vi "Read Glimpse simple.vi"() -> ()   [LabVIEW 2014]
uses:
  4.Other/header ctl/Header file data.ctl
  4.Other/header ctl/Offset table.ctl
  4.Other/header ctl/Offset.ctl
  4.Other/header ctl/file number.ctl
panel:
  out "Header file data":T1 {"Pixel depth" items=["8 bits", "16 bits", "Float", "Complex", "RGB", "HSL"]; "time of 1st frame, \nsec since 1/1/04" format="%.2f"}
  out "size(s)":i32
  out "TTB Array (ms)":u32[](array[numeric])
  out "Array":u32[](array[numeric])
  in  "Data Folder":path
  out "Image":T5(plugin-control)
  out "Width":i32=1200
  out "Height":i32=1920
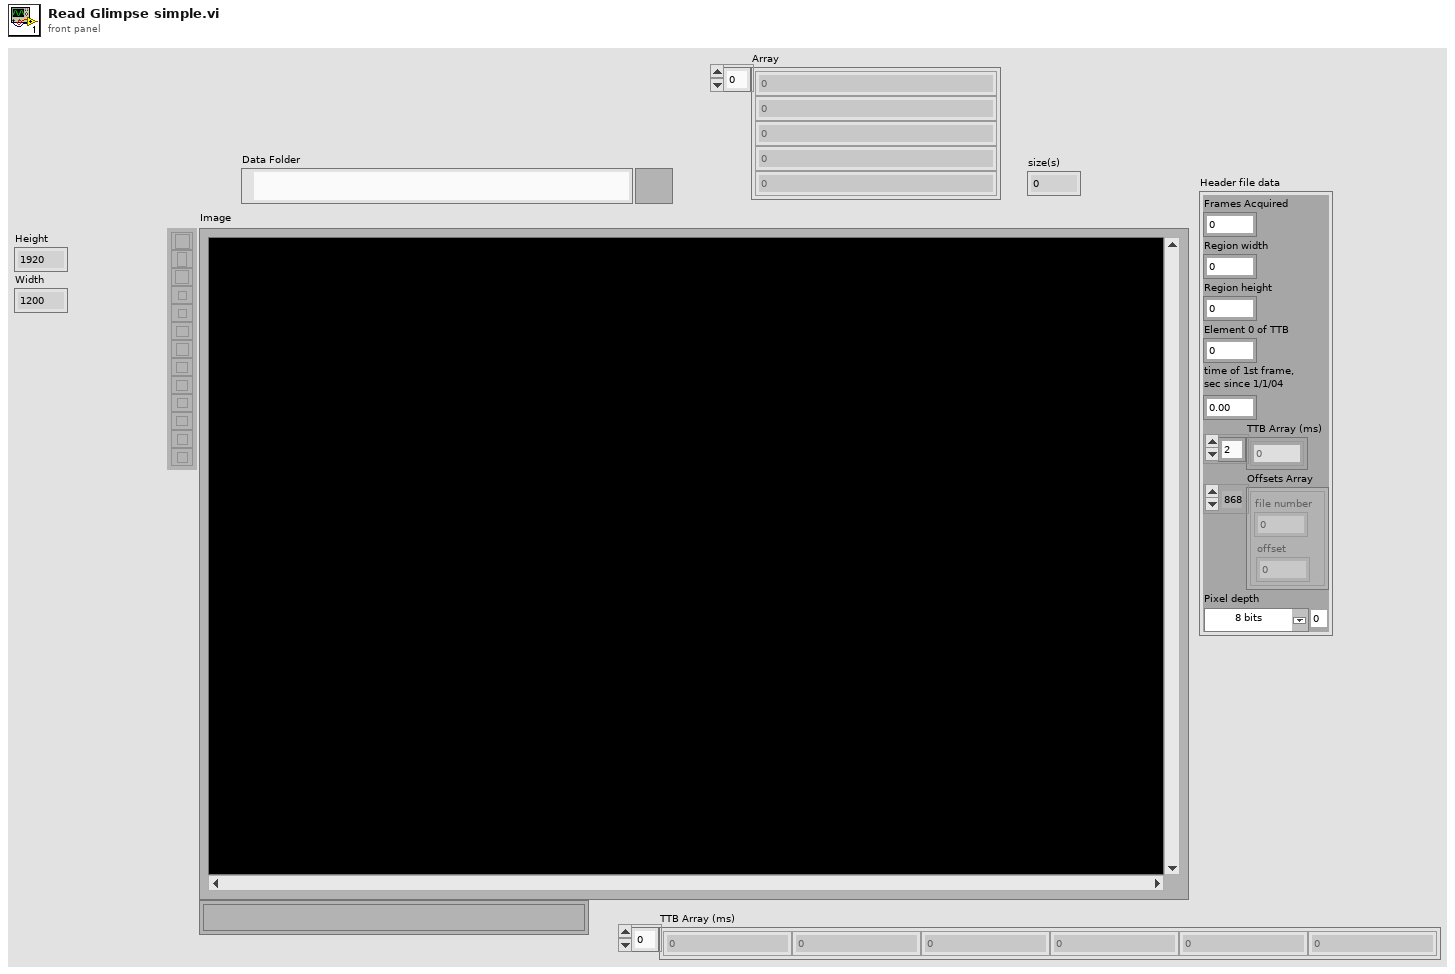
[diagram p1: front panel]
types:
  T1 = typedef "Header file data.ctl" = cluster{"Frames Acquired":u32, "Region width":i32, "Region height":i32, "Element 0 of TTB":u32, "time of 1st frame, \nsec since 1/1/04":dbl, "TTB Array (ms)":u32[], "Offsets Array":T2, "Pixel depth":u32}
  T2 = typedef "Offset table.ctl" = cluster{"offset":T3, "file number":T4}[]
  T3 = typedef "Offset.ctl" = i32
  T4 = typedef "file number.ctl" = u8
  T5 = typedef "IMAQ Image.ctl" = refnum<image>
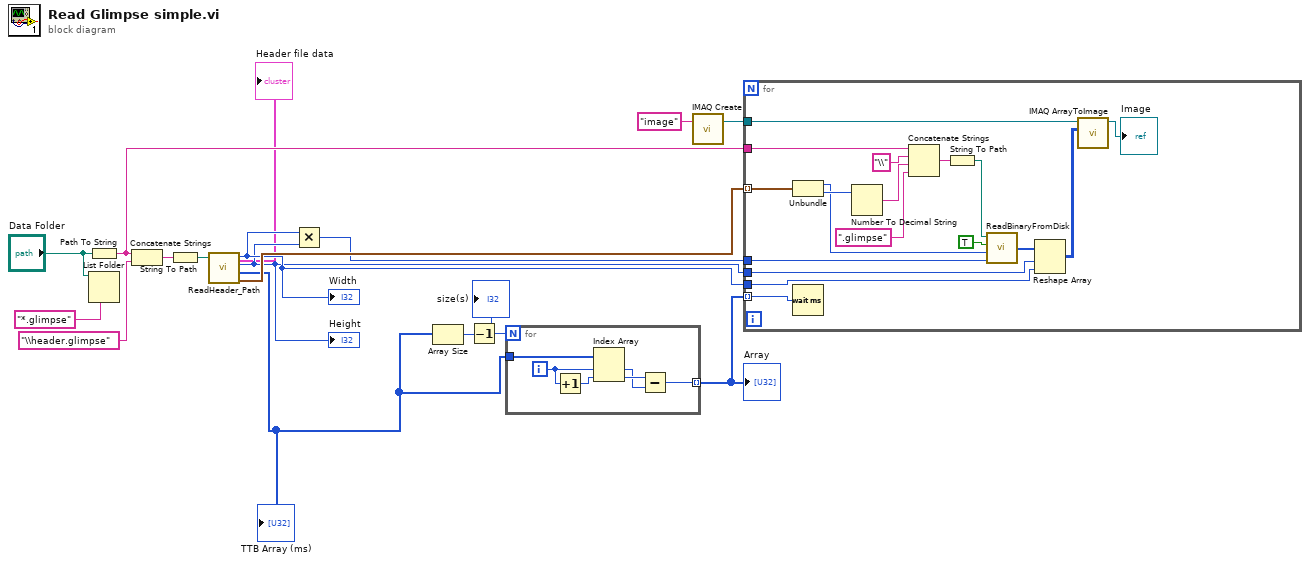
[diagram p0: block diagram]
diagram:
  n1 = Path To String(path="Data Folder") -> (string=w10:string)
  n2 = List Folder(path="Data Folder", pattern="*.glimpse") -> ()  [unwired: 2 in, 4 out]
  n3 = Concatenate Strings(w10, "\\header.glimpse" ("string")) -> (w14:string)
  n4 = String To Path(string=w14) -> (path=w13:path)
  n5 = call "ReadHeader_Path.vi"("datalog path (use dialog)"=w13) -> ("Offsets Array"=w12:T2, "TTB Array (ms)\ntime axis (ms)\n0,1/fs,2/fs,...,n/fs"=w2:u32[], "Region height"=w8:i32, "Header file data"=→"Header file data":T1, "Region width"=w9:i32)  [unwired: 3 in]
  "Height" <- w8
  "Width" <- w9
  "TTB Array (ms)" <- w2
  n6 = Multiply(x=w9, y=w8) -> (x*y=w11:i32)
  n7 = Array Size(array=w2) -> (size(s)=w4:i32)
  "size(s)" <- w4
  n8 = Decrement(x=w4) -> (x-1=w3:i32)
  n9 = for {
    N: w3 -> [_]
    tunnel: w2 -> [w23]
    tunnel: [w18] -> w5 mode=indexing
    i -> [w22]
    n10 = Increment(x=w22) -> (x+1=w21:i32)
    n11 = Index Array(array=w23, index #1=w22, index #2=w21) -> (element #1=w19:u32, element #2=w20:u32)
    n12 = Subtract(x=w20, y=w19) -> (x-y=w18:u32)
  }
  "Array" <- w5
  n13 = call "IMAQ Create"("Image Name"="image") -> ("New Image"=w6:T5)  [unwired: 4 in, 1 out]
  n14 = for {
    tunnel: w12 -> [w40] mode=indexing
    tunnel: w5 -> [w28] mode=indexing
    tunnel: w11 -> [w39]
    tunnel: w10 -> [w38]
    tunnel: w9 -> [w26]
    tunnel: w8 -> [w27]
    tunnel: w6 -> [w29]
    n15 = Unbundle(w40) -> ("offset"=w25:T3, "file number"=w36:T4)
    n16 = Wait (ms)(milliseconds to wait=w28) -> ()  [unwired: 1 out]
    n17 = Number To Decimal String(number=w36) -> (decimal integer string=w35:string)  [unwired: 1 in]
    n18 = Concatenate Strings(w38, "\\" ("string"), w35, ".glimpse" ("string")) -> (w33:string)
    n19 = String To Path(string=w33) -> (path=w24:path)
    n20 = call "ReadBinaryFromDisk.vi"("size to read (count)"=w39, "offset (in bytes) (0)"=w25, "Set Position?"=TRUE, "Read or Write Path"=w24) -> ("data (U8)"=w32:u8[])  [unwired: 1 in, 1 out]
    n21 = Reshape Array(w32, w27, w26) -> (w31:u8[][])
    n22 = call "IMAQ ArrayToImage"("Image Pixels (U8)"=w31, "Image"=w29) -> ("Image Out"=→"Image":T5)  [unwired: 8 in, 1 out]
  }
